vi "PSVCH_Convert Data.vi"(10 "DAQ2ANA":T2[](array[typedef])) -> (2 "VarList":T1)   [LabVIEW 2016]
uses:
  Ctrls/PSVCH_All Channels.ctl
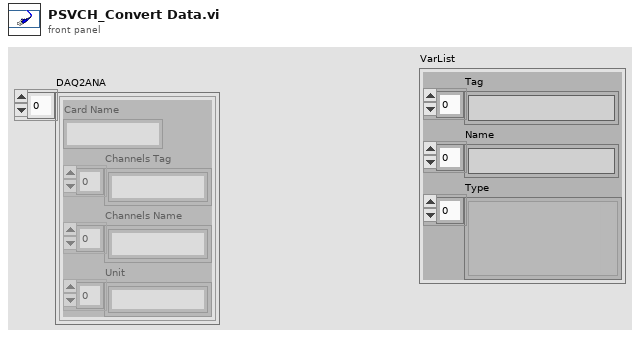
[diagram p1: front panel]
types:
  T1 = cluster{"Tag":string[], "Name":string[], "Type":variant[]}
  T2 = typedef "PSVCH_All Channels.ctl" = cluster{"Card Name":string, "Channels Tag":string[], "Channels Name":string[], "Unit":string[]}
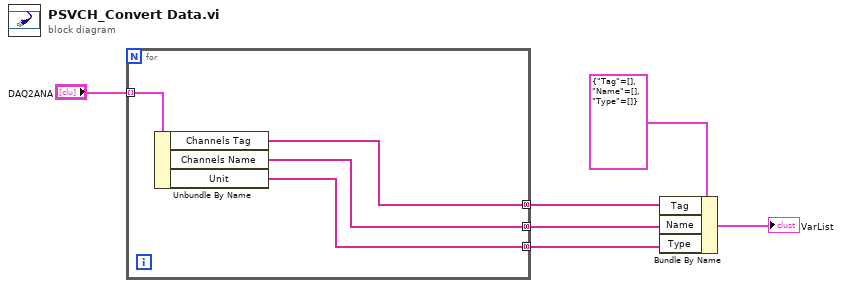
[diagram p0: block diagram]
diagram:
  n1 = for {
    tunnel: "DAQ2ANA" -> [w10] mode=indexing
    tunnel: [w9] -> w4 mode=concatenating
    tunnel: [w8] -> w3 mode=concatenating
    tunnel: [w7] -> w2 mode=concatenating
    n2 = Unbundle By Name(w10) -> ("Channels Tag"=w9:string[], "Channels Name"=w8:string[], "Unit"=w7:string[])
  }
  n3 = Bundle By Name(cluster=T1 {"Tag"=[], "Name"=[], "Type"=[]} ("VarList"), "Tag"=w4, "Name"=w3, "Type"=w2) -> (→"VarList":T1)
